vi "Prepare Log.vi"(8 "error in (no error)":errorcluster, 10 "Prepare Log":T1, 11 "Data Logger Module in":refnum<class "Data Logger Module.lvclass">) -> (0 "error out":errorcluster, 3 "Data Logger Module out":refnum<class "Data Logger Module.lvclass">)   [LabVIEW 2020, in "VolatusData.lvlib" / "Data Logger Module.lvclass"]
uses:
  Data Logger Module.lvclass
  Data Logger Module.lvclass/Data Logger Module.ctl
  Volatus/MessageQ/MessageQ.lvclass
  Logger Ready.ctl
  VolatusData.lvlib
  Prepare Log.ctl
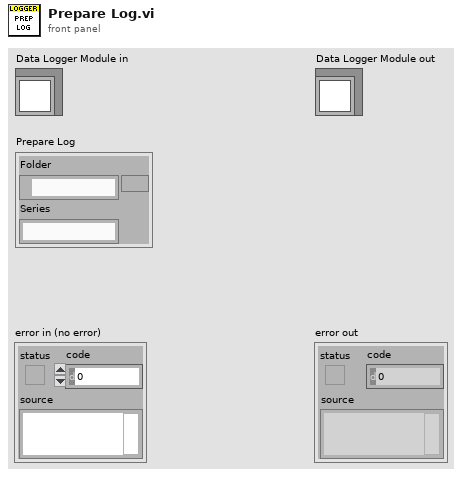
[diagram p1: front panel]
types:
  T1 = typedef "VolatusData.lvlib/Prepare Log.ctl" = cluster{"Folder":path, "Series":string}
  T2 = enum16{"open", "open or create", "create or replace", "create", "open (read-only)"}
  T3 = typedef "VolatusData.lvlib/Logger Ready.ctl" = cluster{"ID":string}
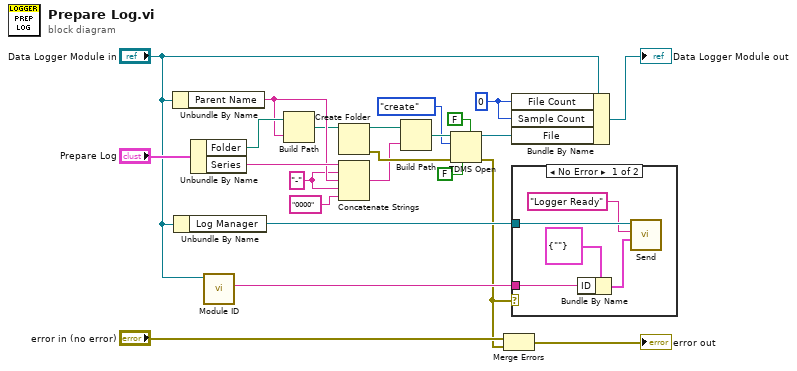
[diagram p0: block diagram]
diagram:
  w13 = 0
  w16 = "-" ("string")
  n1 = Unbundle By Name("Data Logger Module in") -> ("Parent Name"=w18:string)
  n2 = Unbundle By Name("Data Logger Module in") -> ("Log Manager"=w8:refnum<class "MessageQ.lvclass">)
  n3 = Unbundle By Name("Prepare Log") -> ("Folder"=w20:path, "Series"=w19:string)
  n4 = call-dynamic "Module ID.vi"("Data Logger Module in"="Data Logger Module in") -> ("Module ID"=w7:string)  [unwired: 10 in]
  n5 = Build Path(base path=w20, name or relative path=w18) -> (appended path=w17:path)
  n6 = Create Folder(path (use dialog)=w17) -> (created path=w12:path, error out=w23:errorcluster)  [unwired: 2 in, 1 out]
  n7 = Concatenate Strings(w19, w16, w18, w16, "0000" ("string")) -> (w11:string)
  n8 = Build Path(base path=w12, name or relative path=w11) -> (appended path=w6:path)
  n9 = TDMS Open(5:FALSE ("create index file? (T)"), 6:FALSE ("disable buffering? (T)"), 8:w23, 10:T2."create" ("operation (0:open)"), 11:w6) -> (0:w2:errorcluster, 3:w1:refnum<k34>)  [unwired: 2 in]
  n10 = Merge Errors("error in (no error)", w2) -> (→"error out":errorcluster)
  n11 = Bundle By Name(cluster="Data Logger Module in", "File Count"=w13, "Sample Count"=w13, "File"=w1) -> (→"Data Logger Module out":refnum<class "Data Logger Module.lvclass">)
  n12 = case shown="No Error" w2 {
    tunnel: w8 -> [w28 _]
    tunnel: w7 -> [w24 _]
    frame No Error {
      n13 = Bundle By Name(cluster=T3 {"ID"=""} ("Logger Ready"), "ID"=w24) -> (w26:T3)
      n14 = call "Send.vi"("Data"=w26, "ID"="Logger Ready", "MessageQ in"=w28) -> ()  [unwired: 7 in, 2 out]
    }
    frame Error {
    }
  }
